vi "CreateSNRegisterValues.vi"(8 "SerialNo":u16, 9 "Line":u16, 10 "Shift":u16, 11 "Datecode":string) -> (0 "$2C":u32 format="%b", 1 "$2B":u32 format="%b", 2 "$2A":u32 format="%b", 3 "$29":u32 format="%b")   [LabVIEW 2017]
panel:
  out "WeekDay":i32 format="%b"
  out "Year":i32 format="%b"
  out "WeekDay":string
  out "Week":string
  out "Year":string
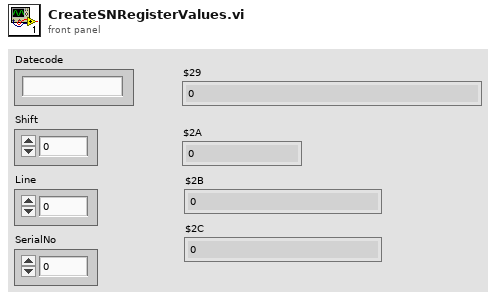
[diagram p1: front panel]
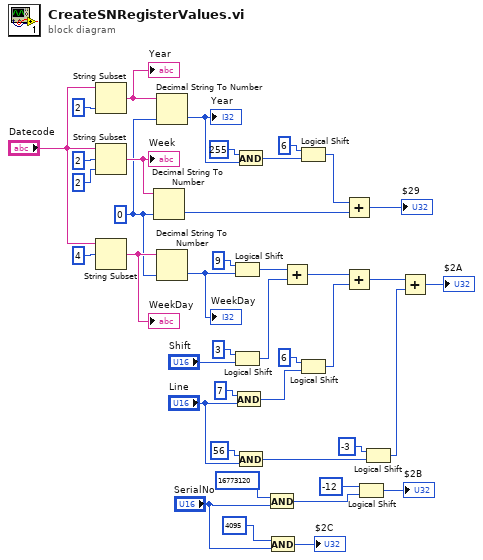
[diagram p0: block diagram]
diagram:
  w33 = u16 0 ("default (0 I32)")
  n1 = String Subset(string="Datecode", length (rest)=2 ("length (rest)")) -> (substring=w36:string)  [unwired: 1 in]
  "Year" <- w36
  n2 = String Subset(string="Datecode", offset (0)=2, length (rest)=2 ("length (rest)")) -> (substring=w35:string)
  "Week" <- w35
  n3 = String Subset(string="Datecode", offset (0)=4) -> (substring=w34:string)  [unwired: 1 in]
  "WeekDay" <- w34
  n4 = Decimal String To Number(string=w35, default (0L)=w33) -> (number=w26:u16)  [unwired: 1 in, 1 out]
  n5 = Decimal String To Number(string=w36, default (0L)=w33) -> (number=w30:u16)  [unwired: 1 in, 1 out]
  "Year" <- w30
  n6 = Decimal String To Number(string=w34, default (0L)=w33) -> (number=w25:u16)  [unwired: 1 in, 1 out]
  "WeekDay" <- w25
  n7 = Logical Shift(y=i16 9, x=w25) -> (x << y=w21:u16)
  n8 = Logical Shift(y=i16 3, x="Shift") -> (x << y=w20:u16)
  n9 = And(x=u8 7, y="Line") -> (x .and. y?=w1:u16)
  n10 = And(x=u16 255 ("y"), y=w30) -> (x .and. y?=w32:u16)
  n11 = And(x=u8 56, y="Line") -> (x .and. y?=w13:u16)
  n12 = And(x=u64 16773120, y="SerialNo") -> (x .and. y?=w6:u64)
  n13 = And(x=u64 4095, y="SerialNo") -> (x .and. y?=→"$2C":u64)
  n14 = Add(x=w21, y=w20) -> (x+y=w15:u16)
  n15 = Logical Shift(y=i16 6, x=w32) -> (x << y=w28:u16)
  n16 = Logical Shift(y=i16 6, x=w1) -> (x << y=w14:u16)
  n17 = Add(x=w28, y=w26) -> (x+y=→"$29":u16)
  n18 = Add(x=w15, y=w14) -> (x+y=w10:u16)
  n19 = Logical Shift(y=i16 -12, x=w6) -> (x << y=→"$2B":u64)
  n20 = Logical Shift(y=i16 -3, x=w13) -> (x << y=w11:u16)
  n21 = Add(x=w10, y=w11) -> (x+y=→"$2A":u16)
